vi "Discretization_DiscretizeAQTaylor.vi"(6 "dT_Seconds":dbl, 9 "ContQ":T1, 10 "ContA":T1, 11 "States":i32) -> (0 "Error":bool, 1 "DiscQ":T1, 3 "DiscA":T1)   [LabVIEW 2019, in "Trajectory_Library.lvlib"]
doc: "Creates a new LINEAR SYSTEM data cluster with the specified values. \n\n\nInputs: \n - XXX -- XXX.\n\nOutputs:\n - XXX -- XXX."
uses:
  Trajectory_Library.lvlib
  <vilib>/Analysis/NI_AALPro.lvlib
  <vilib>/Analysis/7linalg.llb/Real Transpose Matrix.vi
  <vilib>/Analysis/Matrix/NI_Matrix.lvlib
  <vilib>/Analysis/Matrix/Numeric/Add/Add - RM,RM.vi
  <vilib>/Analysis/Matrix/Numeric/Multiply/Multiply - RM,R.vi
  <vilib>/Analysis/NI_AALBase.lvlib
  <vilib>/Analysis/baseanly.llb/Real A x B.vi
  <vilib>/Analysis/Matrix/Datatypes/RealMatrix.ctl
panel:
  # "<States,States>"
  # "<States,States>"
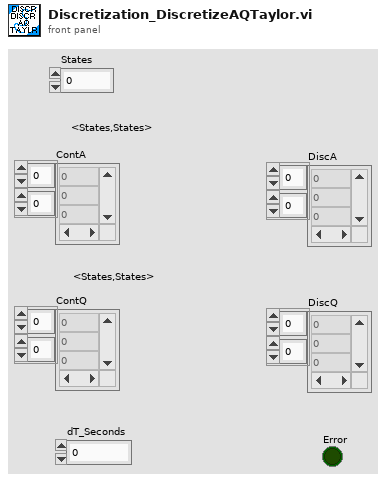
[diagram p1: front panel]
types:
  T1 = typedef "NI_Matrix.lvlib/RealMatrix.ctl" = dbl[][]
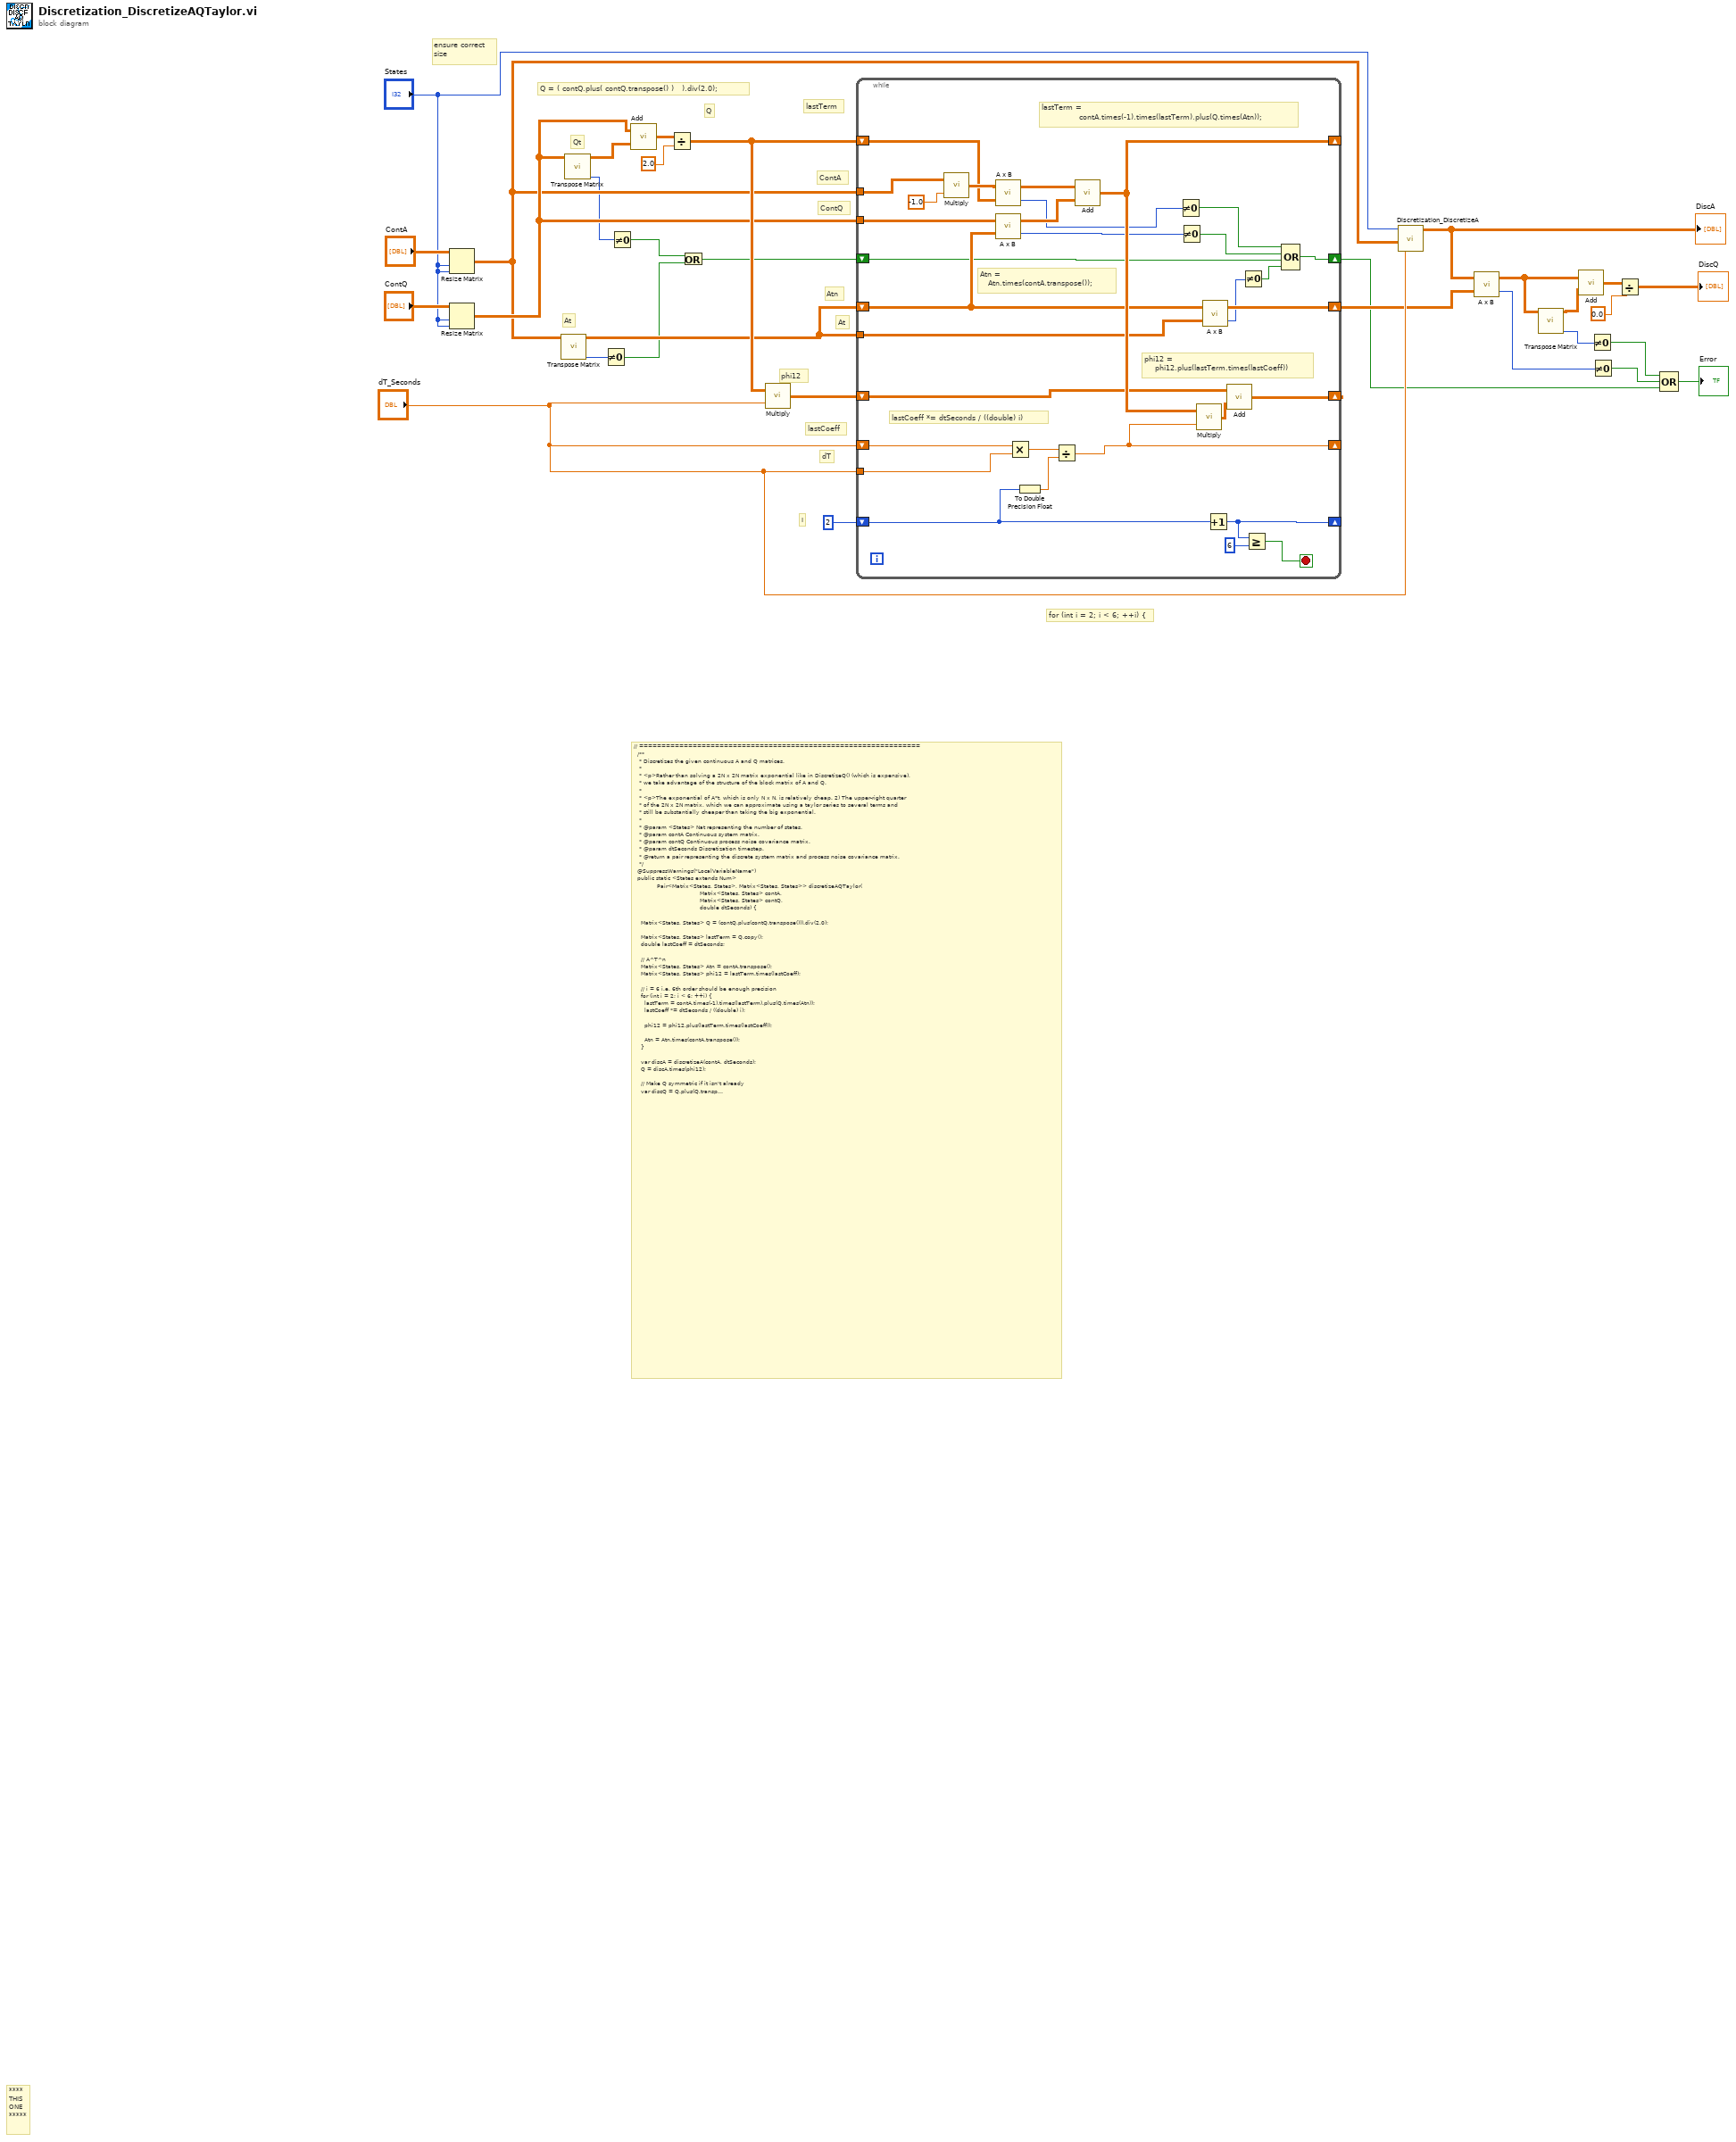
[diagram p0: block diagram]
diagram:
  # "dT"
  # "At"
  # "ContQ"
  # "ContA"
  # "for (int i = 2; i < 6; ++i) {"
  # "Atn"
  # "I"
  # "phi12"
  # "Qt"
  # "At"
  # "lastCoeff"
  # "lastTerm"
  # "Q"
  # "Q = ( contQ.plus( contQ.transpose() )   ).div(2.0);"
  # "// ===============================================================\n  /**\n   * Discretizes the given continuous A and Q matrices.\n   *\n   * <p>Rather than solving a 2N x 2N matrix exponential like in DiscretizeQ() (which is expensive),\n   * we take advantage of the structure of the block matrix of A and Q.\n   *\n   * <p>The exponential of A*t, which is only N x N, is relatively cheap. 2) The upper-right quarter\n   * of the 2N x 2N matrix, which we can approximate using a taylor series to several terms and\n   * still be substantially cheaper than taking the big exponential.\n   *\n   * @param <States> Nat representing the number of states.\n   * @param contA Continuous system matrix.\n   * @param contQ Continuous process noise covariance matrix.\n   * @param dtSeconds Discretization timestep.\n   * @return a pair representing the discrete system matrix and process noise covariance matrix.\n   */\n  @SuppressWarnings(\"LocalVariableName\")\n  public static <States extends Num>\n             Pair<Matrix<States, States>, Matrix<States, States>> discretizeAQTaylor(\n                                     Matrix<States, States> contA, \n                                     Matrix<States, States> contQ, \n                                     double dtSeconds) {\n\n    Matrix<States, States> Q = (contQ.plus(contQ.transpose())).div(2.0);\n\n    Matrix<States, States> lastTerm = Q.copy();\n    double lastCoeff = dtSeconds;\n\n    // A^T^n\n    Matrix<States, States> Atn = contA.transpose();\n    Matrix<States, States> phi12 = lastTerm.times(lastCoeff);\n\n    // i = 6 i.e. 6th order should be enough precision\n    for (int i = 2; i < 6; ++i) {\n      lastTerm = contA.times(-1).times(lastTerm).plus(Q.times(Atn));\n      lastCoeff *= dtSeconds / ((double) i);\n\n      phi12 = phi12.plus(lastTerm.times(lastCoeff));\n\n      Atn = Atn.times(contA.transpose());\n    }\n\n    var discA = discretizeA(contA, dtSeconds);\n    Q = discA.times(phi12);\n\n    // Make Q symmetric if it isn't already\n    var discQ = Q.plus(Q.transpose()).div(2.0);\n\n    return new Pair<>(discA, discQ);\n  }"
  # "ensure correct\nsize"
  # "****\nTHIS\nONE\n*****"
  n1 = Resize Matrix(1:"States", 2:"States", 4:"ContA") -> (0:w21:T1)
  n2 = Resize Matrix(1:"States", 2:"States", 4:"ContQ") -> (0:w24:T1)
  n3 = call-poly <vilib>:"Transpose Matrix.vi"("Input Matrix"=w21) -> ("error"=w11:i32, "Matrix Transpose"=w22:T1)  [unwired: 9 in]
  n4 = call-poly <vilib>:"Transpose Matrix.vi"("Input Matrix"=w24) -> ("error"=w10:i32, "Matrix Transpose"=w29:T1)  [unwired: 9 in]
  n5 = Not Equal To 0?(x=w11) -> (x != 0?=w8:bool)
  n6 = Not Equal To 0?(x=w10) -> (x != 0?=w9:bool)
  n7 = call-poly <vilib>:"Add.vi"("Real Matrix B"=w29, "Real Matrix A"=w24) -> ("A + B"=w28:T1)
  n8 = Divide(x=w28, y=2.0) -> (x/y=w26:T1)
  n9 = Or(x=w9, y=w8) -> (x .or. y?=w7:bool)
  n10 = call-poly <vilib>:"Multiply.vi"("Real Scalar c"="dT_Seconds", "Real Matrix A"=w26) -> ("A * c"=w23:T1)
  n11 = while {
    shift-right: [w51] -> _
    shift-left: w26 -> [w60]
    shift-right: [w52] -> _
    shift-left: "dT_Seconds" -> [w56]
    shift-right: [w42] -> _
    shift-left: 2 -> [w43]
    tunnel: w21 -> [w44]
    tunnel: w24 -> [w59]
    tunnel: "dT_Seconds" -> [w55]
    shift-right: [w48] -> _
    shift-left: w23 -> [w50]
    shift-right: [w45] -> w17
    shift-left: w22 -> [w47]
    tunnel: w22 -> [w46]
    shift-right: [w39] -> w4
    shift-left: w7 -> [w38]
    stop <- w40 stop-if-true
    # "Atn = \n   Atn.times(contA.transpose());"
    # "phi12 = \n    phi12.plus(lastTerm.times(lastCoeff))"
    # "lastCoeff *= dtSeconds / ((double) i)"
    # "lastTerm = \n              contA.times(-1).times(lastTerm).plus(Q.times(Atn));"
    n12 = call-poly <vilib>:"Multiply.vi"("Real Scalar c"=-1.0, "Real Matrix A"=w44) -> ("A * c"=w61:T1)
    n13 = call-poly <vilib>:"A x B.vi"("B"=w60, "A"=w61) -> ("error"=w37:i32, "A x B"=w58:T1)
    n14 = call-poly <vilib>:"A x B.vi"("B"=w47, "A"=w59) -> ("error"=w36:i32, "A x B"=w57:T1)
    n15 = Multiply(x=w56, y=w55) -> (x*y=w54:dbl)
    n16 = To Double Precision Float(number=w43) -> (double precision float=w53:dbl)
    n17 = Divide(x=w54, y=w53) -> (x/y=w52:dbl)
    n18 = call-poly <vilib>:"Add.vi"("Real Matrix B"=w57, "Real Matrix A"=w58) -> ("A + B"=w51:T1)
    n19 = Not Equal To 0?(x=w37) -> (x != 0?=w32:bool)
    n20 = Not Equal To 0?(x=w36) -> (x != 0?=w33:bool)
    n21 = call-poly <vilib>:"Multiply.vi"("Real Scalar c"=w52, "Real Matrix A"=w51) -> ("A * c"=w49:T1)
    n22 = call-poly <vilib>:"A x B.vi"("B"=w46, "A"=w47) -> ("error"=w34:i32, "A x B"=w45:T1)
    n23 = Increment(x=w43) -> (x+1=w42:i32)
    n24 = call-poly <vilib>:"Add.vi"("Real Matrix B"=w49, "Real Matrix A"=w50) -> ("A + B"=w48:T1)
    n25 = Not Equal To 0?(x=w34) -> (x != 0?=w35:bool)
    n26 = Greater Or Equal?(x=w42, y=6) -> (x >= y?=w40:bool)
    n27 = Compound Arithmetic op=OR(w32, w33, w38, w35) -> (w39:bool)
  }
  n28 = call "Discretization_DiscretizeA.vi"("dT_Seconds"="dT_Seconds", "ContA"=w21, "States"="States") -> ("DiscA"=w18:T1)  [unwired: 7 in, 1 out]
  "DiscA" <- w18
  n29 = call-poly <vilib>:"A x B.vi"("B"=w17, "A"=w18) -> ("error"=w5:i32, "A x B"=w16:T1)
  n30 = call-poly <vilib>:"Transpose Matrix.vi"("Input Matrix"=w16) -> ("error"=w6:i32, "Matrix Transpose"=w15:T1)  [unwired: 9 in]
  n31 = call-poly <vilib>:"Add.vi"("Real Matrix B"=w15, "Real Matrix A"=w16) -> ("A + B"=w14:T1)
  n32 = Not Equal To 0?(x=w6) -> (x != 0?=w2:bool)
  n33 = Not Equal To 0?(x=w5) -> (x != 0?=w3:bool)
  n34 = Divide(x=w14, y=0.0) -> (x/y=→"DiscQ":T1)
  n35 = Compound Arithmetic op=OR(w2, w3, w4) -> (→"Error":bool)
